vi "cent$.vi"(6 "Switch o' Suffering":bool, 11 "Cents In":dbl) -> (3 "Dollar String":string)   [LabVIEW 2016]
uses:
  <vilib>/gmath/NI_Gmath.lvlib
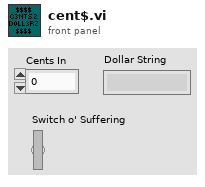
[diagram p1: front panel]
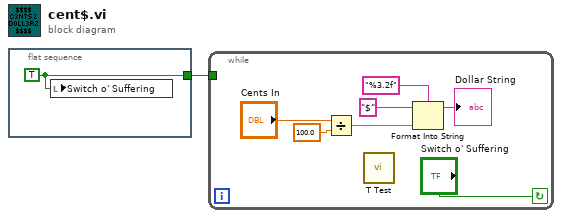
[diagram p0: block diagram]
diagram:
  n1 = flat-sequence {
    tunnel: [w2] -> w1
    frame #0 {
      w2 = TRUE
      n2 = local write "Switch o' Suffering"(w2) -> ()
    }
  }
  n3 = while {
    tunnel: w1 -> [_]
    stop <- "Switch o' Suffering" continue-if-true
    n4 = Divide(x="Cents In", y=100.0) -> (x/y=w6:dbl)
    n5 = call <vilib>:"T Test.vi"() -> ()  [unwired: 7 in, 5 out]
    n6 = Format Into String(format string="%3.2f", initial string="$", w6) -> (resulting string=→"Dollar String":string)  [unwired: 1 in, 1 out]
  }
